vi "Initialize Device Core.vi"(8 "error in (no error)":errorcluster, 9 "Reset (F)":bool, 10 "Resource Name":string, 11 "BNT_ULx-MCSV-DOPWM in":refnum<class "BNT_ULx-MCSV-DOPWM.lvclass">) -> (0 "error out":errorcluster, 3 "BNT_ULx-MCSV-DOPWM out":refnum<class "BNT_ULx-MCSV-DOPWM.lvclass">)   [LabVIEW 2020, in "BNT_ULx.lvlib" / "BNT_ULx-MCSV-DOPWM.lvclass"]
doc: "Initialize device driver."
uses:
  BNT_ULx-MCSV-DOPWM.lvclass
  C:/User/Brand/LVP/CSPP/CSPP-Template/Packages/BNT_ULx/BNT_ULx-MCSV/BNT_ULx-MCSV/BNT_ULx-MCSV.lvclass
  BNT_ULx-MCSV/BNT_ULx-MCSV.lvclass/BNT_ULx-MCSV.ctl
  BNT_ULx-MCSV-DOPWM.lvclass/BNT_ULx-MCSV-DOPWM.ctl
  BNT_ULx-MCSV/BNT_ULx-MCSV.lvclass
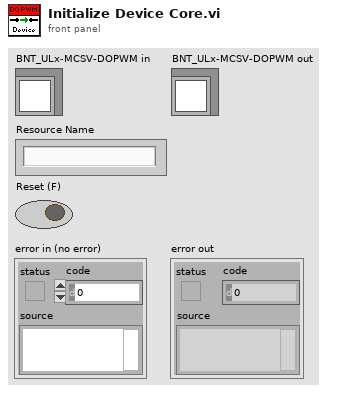
[diagram p1: front panel]
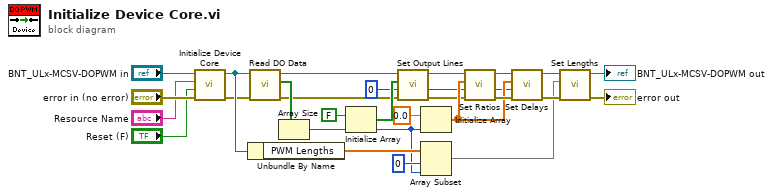
[diagram p0: block diagram]
diagram:
  w5 = 0 ("Start Index")
  n1 = call-parent "Initialize Device Core.vi"("error in (no error)"="error in (no error)", "Reset (F)"="Reset (F)", "Resource Name"="Resource Name", "BNT_ULx-MCSV in"="BNT_ULx-MCSV-DOPWM in") -> ("error out"=w7:errorcluster, "BNT_ULx-MCSV out"=w8:refnum<class "BNT_ULx-MCSV-DOPWM.lvclass">)  [unwired: 6 in]
  n2 = Unbundle By Name(w8) -> ("PWM Lengths"=w17:dbl[unit][])
  n3 = call "Read DO Data.vi"("error in (no error)"=w7, "BNT_ULx-MCSV in"=w8) -> ("error out"=w2:errorcluster, "DO Data"=w9:bool[], "BNT_ULx-MCSV out"=w4:refnum<class "BNT_ULx-MCSV-DOPWM.lvclass">)  [unwired: 7 in]
  n4 = Array Size(array=w9) -> (size(s)=w15:i32)
  n5 = Initialize Array(FALSE, w15) -> (w6:bool[])
  n6 = call "Set Output Lines.vi"("Error In"=w2, "Start Index"=w5, "DO Lines"=w6, "BNT_ULx-MCSV in"=w4) -> ("Error Out"=w1:errorcluster, "BNT_ULx-MCSV out"=w3:refnum<class "BNT_ULx-MCSV-DOPWM.lvclass">)  [unwired: 6 in]
  n7 = Initialize Array(0.0, w15) -> (w18:dbl[])
  n8 = Array Subset(array=w17, index=0, length=w15) -> (w10:dbl[unit][])
  n9 = call "Set Ratios.vi"("error in"=w1, "Start Index"=w5, "PWM Ratios"=w18, "BNT_ULx-MCSV-DOPWM in"=w3) -> ("error out"=w20:errorcluster, "BNT_ULx-MCSV-DOPWM out"=w21:refnum<class "BNT_ULx-MCSV-DOPWM.lvclass">)  [unwired: 6 in]
  n10 = call "Set Delays.vi"("error in"=w20, "Start Index"=w5, "PWM Delays"=w18, "BNT_ULx-MCSV-DOPWM in"=w21) -> ("error out"=w12:errorcluster, "BNT_ULx-MCSV-DOPWM out"=w14:refnum<class "BNT_ULx-MCSV-DOPWM.lvclass">)  [unwired: 6 in]
  n11 = call "Set Lengths.vi"("error in"=w12, "PWM Lengths"=w10, "BNT_ULx-MCSV-DOPWM in"=w14) -> ("error out"=→"error out":errorcluster, "BNT_ULx-MCSV-DOPWM out"=→"BNT_ULx-MCSV-DOPWM out":refnum<class "BNT_ULx-MCSV-DOPWM.lvclass">)  [unwired: 7 in]
